vi "getGroupDof.vi"(7 "Input DOF":dbl[](array[numeric]), 8 "error in (no error)":errorcluster, 9 "Group Length":i32, 10 "Start Index":i32, 11 "OptCtrl in":refnum<class "OptCtrl.lvclass">) -> (0 "error out":errorcluster, 2 "DOF":dbl[](array[numeric]), 3 "OptCtrl out":refnum<class "OptCtrl.lvclass">)   [LabVIEW 2016, in "OfcFunc.lvlib" / "OptCtrl.lvclass"]
doc: "Get the degree of freedom (DOF) of specific group based on the start index and length. If there is no input DOF, the output will be the aggregated DOF (state - state0)."
uses:
  OptCtrl.lvclass
  OptCtrl.lvclass/OptCtrl.ctl
  MatOper/getSubArray1D.vi
  MatOper/MatOper.lvclass
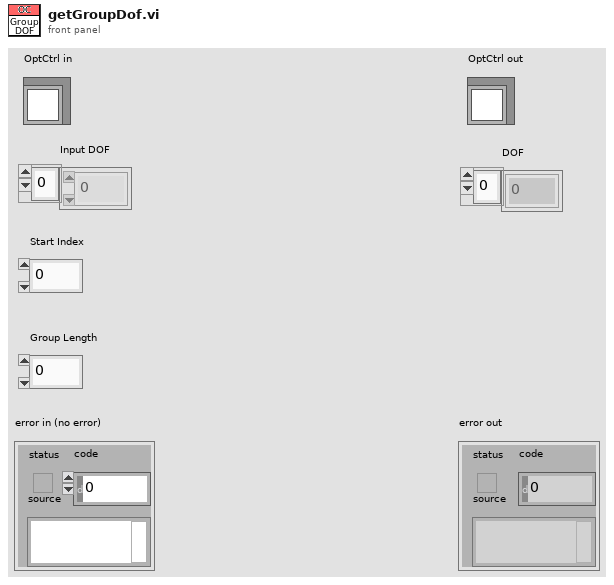
[diagram p1: front panel]
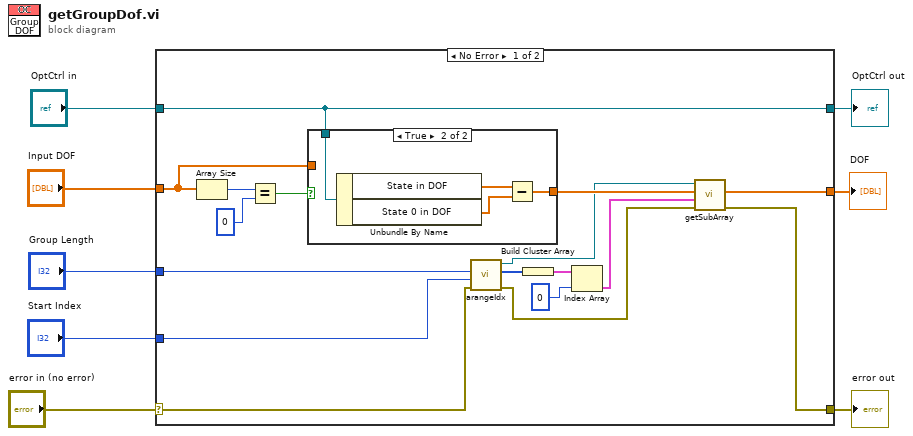
[diagram p0: block diagram]
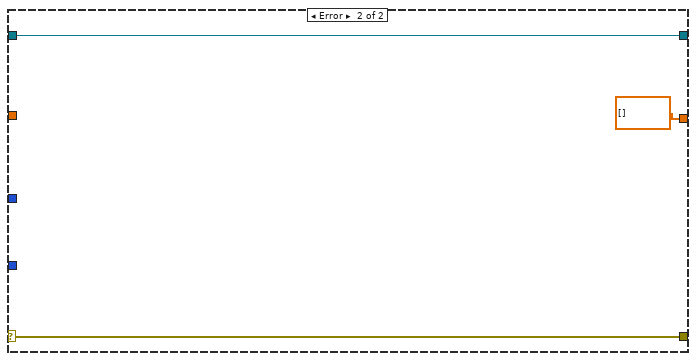
[diagram p3: hidden frame]
diagram:
  n1 = case shown="No Error" "error in (no error)" {
    selector: "error in (no error)" -> [w11 w33]
    tunnel: [w25 w33] -> w7
    tunnel: [w14 w32] -> w5
    tunnel: "OptCtrl in" -> [w14 w32]
    tunnel: [w20 dbl[] [] ("Sub-Array")] -> w4
    tunnel: "Group Length" -> [w19 _]
    tunnel: "Start Index" -> [w18 _]
    tunnel: "Input DOF" -> [w12 _]
    frame No Error {
      n2 = Array Size(array=w12) -> (size(s)=w17:i32)
      n3 = Equal?(x=w17, y=0) -> (x = y?=w15:bool)
      n4 = case shown="True" w15 {
        tunnel: w14 -> [_ w28]
        tunnel: [w26 w27] -> w13
        tunnel: w12 -> [w26 _]
        frame False {
        }
        frame True {
          n5 = Unbundle By Name(w28) -> ("State in DOF"=w30:dbl[], "State 0 in DOF"=w29:dbl[])
          n6 = Subtract(x=w30, y=w29) -> (x-y=w27:dbl[])
        }
      }
      n7 = call "arangeIdx.vi"("error in (no error)"=w11, "Offset"=w18, "Number"=w19) -> ("error out"=w10:errorcluster, "Idx Array"=w22:i32[], "MatOper out"=w9:refnum<class "MatOper.lvclass">)  [unwired: 6 in]
      n8 = Build Cluster Array(w22) -> (w24:cluster{"Idx Array":i32[]}[])
      n9 = Index Array(array=w24, index=0) -> (element=w21:cluster{"Idx Array":i32[]})
      n10 = call-poly "getSubArray.vi"("error in (no error)"=w10, "Index Array Cluster"=w21, "1D Array"=w13, "MatOper in"=w9) -> ("error out"=w25:errorcluster, "Sub-Array"=w20:dbl[])  [unwired: 5 in, 1 out]
    }
    frame Error {
    }
  }
  "error out" <- w7
  "OptCtrl out" <- w5
  "DOF" <- w4
